vi "toCompiledXml.vi"(8 "error in (no error)":errorcluster, 11 "ScriptEventList in":refnum<class "ScriptEventList.lvclass">) -> (0 "error out":errorcluster, 2 "compiledXml":refnum<class "xmlNode.lvclass">, 3 "ScriptEventList out":refnum<class "ScriptEventList.lvclass">)   [LabVIEW 2009, in "Tools.lvlib" / "Scripting.lvlib" / "ScriptEventList.lvclass"]
uses:
  ScriptEventList.lvclass
  xmlNode/xmlNode.lvclass
  ScriptEventList.lvclass/ScriptEventList.ctl
  ScriptEvent.lvclass
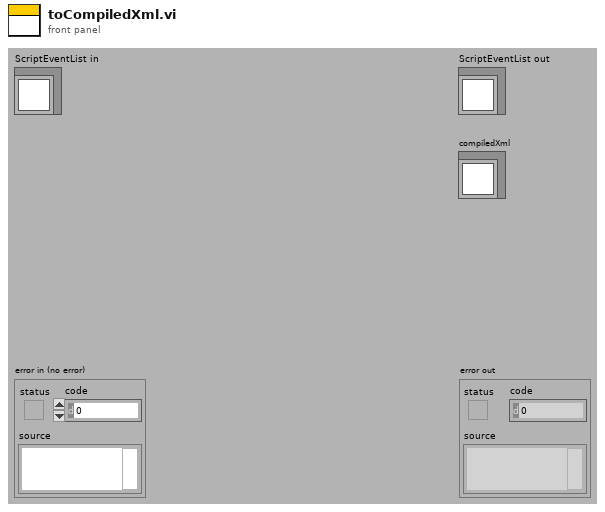
[diagram p1: front panel]
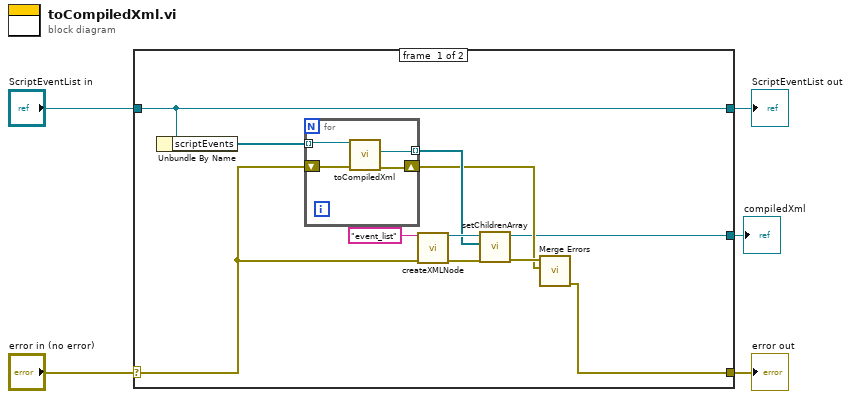
[diagram p0: block diagram]
diagram:
  n1 = case shown="No Error" "error in (no error)" {
    selector: "error in (no error)" -> [w8 w22]
    tunnel: [w7 w22] -> w4
    tunnel: [w12 w21] -> w2
    tunnel: "ScriptEventList in" -> [w12 w21]
    tunnel: [w6 _] -> w1
    frame #0 {
      n2 = Unbundle By Name(w12) -> ("scriptEvents"=w11:refnum<class "ScriptEvent.lvclass">[])
      n3 = for {
        tunnel: w11 -> [w19] mode=indexing
        shift-right: [w17] -> w9
        shift-left: w8 -> [w20]
        tunnel: [w18] -> w10 mode=indexing
        n4 = call-dynamic "toCompiledXml.vi"("error in (no error)"=w20, "ScriptEvent in"=w19) -> ("error out"=w17:errorcluster, "compiledXML"=w18:refnum<class "xmlNode.lvclass">)  [unwired: 7 in, 1 out]
      }
      n5 = call "createXMLNode.vi"("error in (no error)"=w8, "name"="event_list") -> ("error out"=w15:errorcluster, "xmlNode out"=w16:refnum<class "xmlNode.lvclass">)  [unwired: 8 in]
      n6 = call-dynamic "setChildrenArray.vi"("error in (no error)"=w15, "Children"=w10, "xmlNode.lvclass in"=w16) -> ("error out"=w13:errorcluster, "xmlNode.lvclass out"=w6:refnum<class "xmlNode.lvclass">)  [unwired: 7 in]
      n7 = call <vilib>:"Merge Errors.vi"("error in 2 (no error)"=w9, "error in 1 (no error)"=w13) -> ("error out"=w7:errorcluster)  [unwired: 5 in]
    }
    frame #1 {
    }
  }
  "error out" <- w4
  "ScriptEventList out" <- w2
  "compiledXml" <- w1
